vi "VI Tree.vi"   [LabVIEW 2016, in "APT 300XAC Series.lvlib"]
doc: "This instrument driver supports the Associated Power Technologies 300XAC Series Automated AC Power Source\".\n<B>Model Number</B> : 310XAC, 320XAC, 340XAC, 360XAC.\n\nThe VI Tree displays all the user-callable VIs of the instrument driver in an organized table.\n\nAC Range Program mode:\nValue = 0-8; 0=F, 1=A, 2=P, 3=Q, 4=CF, 5=AP, 6=VA, 7=PF, 8=CYCLE\n\nAC Range Manual mode\nValue = 0-7; 0=F, 1=A, 2=P, 3=Q, 4=CF, 5=AP, 6=VA, 7=PF\n\nDC Range Program mode\nValue = 1,2,8; 1=A, 2=P, 8=CYCLE\n\nDC Range Manual mode\nValue = 1,2,8; 1=A, 2=P\n\n\nCreated By:\nAssociated Power Technologies, Inc."
uses:
  APT 300XAC Series.lvlib
  Data/Read Test Data (AC Parallel L1N Program Mode).vi
  Data/Read Test Data (AC Parallel L1N Manual Mode).vi
  Data/Read Step Data (Parallel L1N Manual Mode).vi
  Data/Read Test Data (DC Parallel L1N Program Mode).vi
  Data/Read Test Data (DC Parallel L1N Manual Mode).vi
  Data/Read Step Data (DC Parallel L1N Program Mode).vi
  Data/Read Step Data (DC Parallel L1N Manual Mode).vi
  Data/Read (Voltage).vi
  Data/Read Step Data (AC Total Program Mode).vi
  Data/Read Test Data (AC Program Mode).vi
  Data/Read Step Data (AC Parallel L1N Program Mode).vi
  Data/Read Step Data (AC Polyphase Total Program Mode).vi
  Data/Read Test Data (AC Phase A Program Mode).vi
  Data/Read Test Data (AC Phase A Manual Mode).vi
  Data/Read Step Data (AC Phase A Program Mode).vi
panel:
  # "Associated Power Technologies, Inc. \n1142 S. Diamond Bar Blvd # 106 \nDiamond Bar , CA 91765 \n\nToll Free:  1-877-322-7693\nPhone:      1-909-860-1646\nFax:          1-909-860-2727\nEmail:        info@aspowertechnologies.com"
  # "Please see diagram for APT300XAC Driver VI Tree"
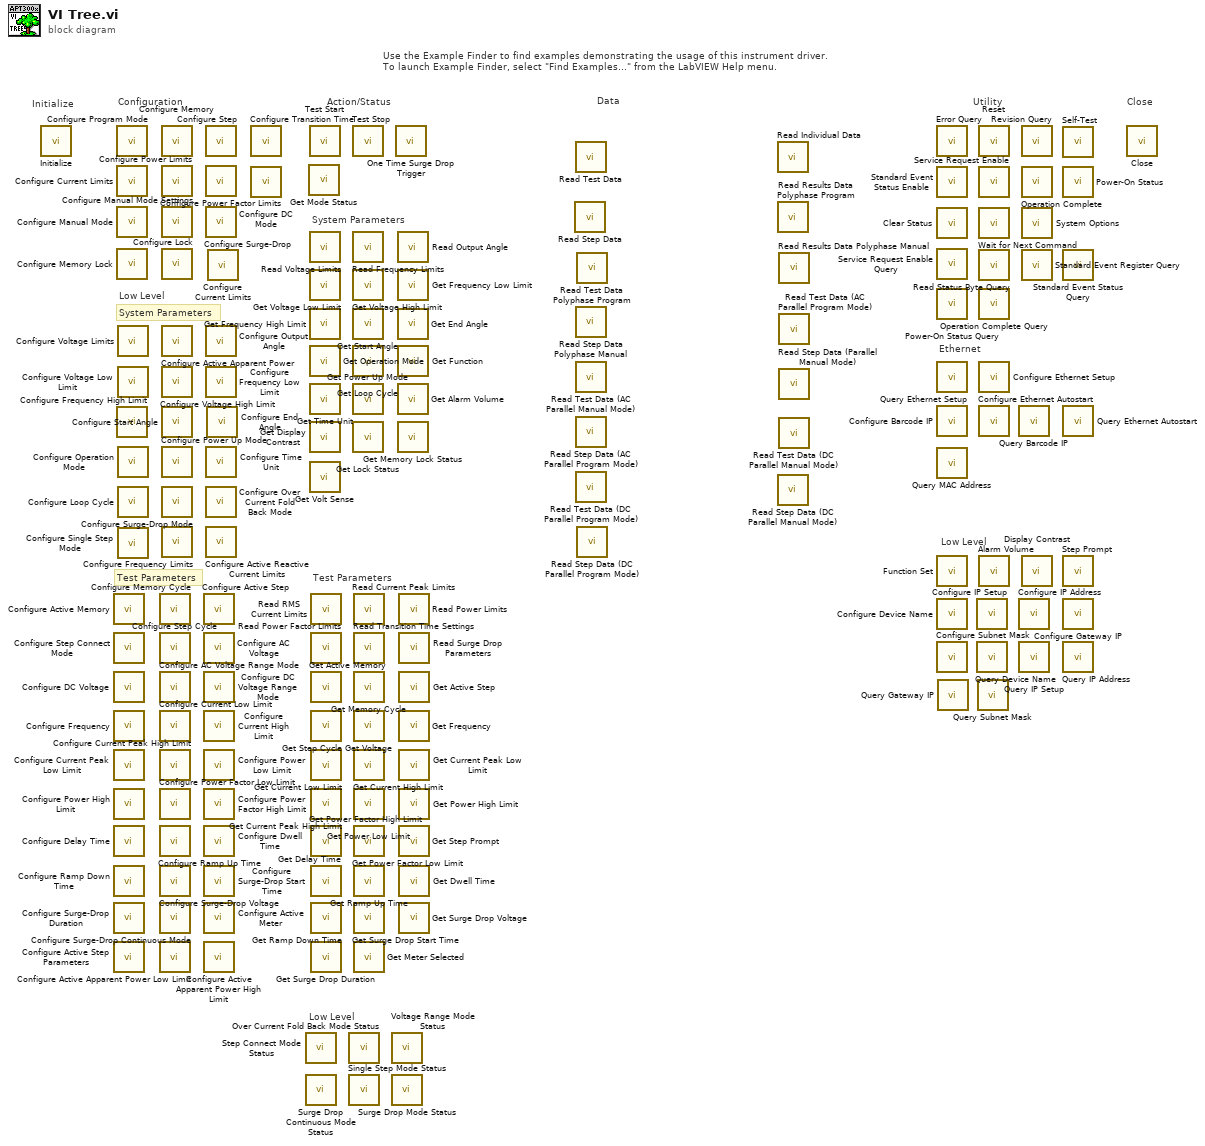
[diagram p0: block diagram]
diagram:
  # "Test Parameters"
  # "System Parameters"
  # "Low Level"
  # "Ethernet"
  # "Low Level"
  # "Use the Example Finder to find examples demonstrating the usage of this instrument driver.\nTo launch Example Finder, select \"Find Examples...\" from the LabVIEW Help menu."
  # "Test Parameters"
  # "System Parameters"
  # "Low Level"
  # "Configuration"
  # "Utility"
  # "Data"
  # "Action/Status"
  # "Close"
  # "Initialize"
  n1 = call "Initialize.vi"() -> ()  [unwired: 14 in, 2 out]
  n2 = call "Configure Active Memory.vi"() -> ()  [unwired: 14 in, 2 out]
  n3 = call "Configure Step Connect Mode.vi"() -> ()  [unwired: 14 in, 2 out]
  n4 = call "Configure DC Voltage.vi"() -> ()  [unwired: 14 in, 2 out]
  n5 = call "Configure Frequency.vi"() -> ()  [unwired: 14 in, 2 out]
  n6 = call "Configure Current Peak Low Limit.vi"() -> ()  [unwired: 14 in, 2 out]
  n7 = call "Configure Power High Limit.vi"() -> ()  [unwired: 14 in, 2 out]
  n8 = call "Configure Delay Time.vi"() -> ()  [unwired: 14 in, 2 out]
  n9 = call "Configure Ramp Down Time.vi"() -> ()  [unwired: 14 in, 2 out]
  n10 = call "Configure Surge-Drop Duration.vi"() -> ()  [unwired: 14 in, 2 out]
  n11 = call "Configure Active Step Parameters.vi"() -> ()  [unwired: 14 in, 2 out]
  n12 = call "Configure Program Mode.vi"() -> ()  [unwired: 14 in, 2 out]
  n13 = call "Configure Current Limits.vi"() -> ()  [unwired: 14 in, 2 out]
  n14 = call "Configure Manual Mode.vi"() -> ()  [unwired: 14 in, 2 out]
  n15 = call "Configure Memory Lock.vi"() -> ()  [unwired: 14 in, 2 out]
  n16 = call "Configure Frequency High Limit.vi"() -> ()  [unwired: 14 in, 2 out]
  n17 = call "Configure Voltage Limits.vi"() -> ()  [unwired: 14 in, 2 out]
  n18 = call "Configure Voltage Low Limit.vi"() -> ()  [unwired: 14 in, 2 out]
  n19 = call "Configure Operation Mode.vi"() -> ()  [unwired: 14 in, 2 out]
  n20 = call "Configure Loop Cycle.vi"() -> ()  [unwired: 14 in, 2 out]
  n21 = call "Configure Single Step Mode.vi"() -> ()  [unwired: 14 in, 2 out]
  n22 = call "Configure Memory Cycle.vi"() -> ()  [unwired: 14 in, 2 out]
  n23 = call "Configure Step Cycle.vi"() -> ()  [unwired: 14 in, 2 out]
  n24 = call "Configure AC Voltage Range Mode.vi"() -> ()  [unwired: 14 in, 2 out]
  n25 = call "Configure Current Low Limit.vi"() -> ()  [unwired: 14 in, 2 out]
  n26 = call "Configure Current Peak High Limit.vi"() -> ()  [unwired: 14 in, 2 out]
  n27 = call "Configure Power Factor Low Limit.vi"() -> ()  [unwired: 14 in, 2 out]
  n28 = call "Configure Ramp Up Time.vi"() -> ()  [unwired: 14 in, 2 out]
  n29 = call "Configure Surge-Drop Voltage.vi"() -> ()  [unwired: 14 in, 2 out]
  n30 = call "Configure Surge-Drop Continuous Mode.vi"() -> ()  [unwired: 14 in, 2 out]
  n31 = call "Configure Active Apparent Power Low Limit.vi"() -> ()  [unwired: 14 in, 2 out]
  n32 = call "Configure Memory.vi"() -> ()  [unwired: 14 in, 2 out]
  n33 = call "Configure Power Limits.vi"() -> ()  [unwired: 14 in, 2 out]
  n34 = call "Configure Manual Mode Settings.vi"() -> ()  [unwired: 14 in, 2 out]
  n35 = call "Configure Lock.vi"() -> ()  [unwired: 14 in, 2 out]
  n36 = call "Configure Active Apparent Power.vi"() -> ()  [unwired: 14 in, 2 out]
  n37 = call "Configure Voltage High Limit.vi"() -> ()  [unwired: 14 in, 2 out]
  n38 = call "Configure Start Angle.vi"() -> ()  [unwired: 14 in, 2 out]
  n39 = call "Configure Power Up Mode.vi"() -> ()  [unwired: 14 in, 2 out]
  n40 = call "Configure Surge-Drop Mode.vi"() -> ()  [unwired: 14 in, 2 out]
  n41 = call "Configure Frequency Limits.vi"() -> ()  [unwired: 14 in, 2 out]
  n42 = call "Configure Active Step.vi"() -> ()  [unwired: 14 in, 2 out]
  n43 = call "Configure AC Voltage.vi"() -> ()  [unwired: 14 in, 2 out]
  n44 = call "Configure DC Voltage Range Mode.vi"() -> ()  [unwired: 14 in, 2 out]
  n45 = call "Configure Current High Limit.vi"() -> ()  [unwired: 14 in, 2 out]
  n46 = call "Configure Power Low Limit.vi"() -> ()  [unwired: 14 in, 2 out]
  n47 = call "Configure Power Factor High Limit.vi"() -> ()  [unwired: 14 in, 2 out]
  n48 = call "Configure Dwell Time.vi"() -> ()  [unwired: 14 in, 2 out]
  n49 = call "Configure Surge-Drop Start Time.vi"() -> ()  [unwired: 14 in, 2 out]
  n50 = call "Configure Active Meter.vi"() -> ()  [unwired: 14 in, 2 out]
  n51 = call "Configure Active Apparent Power High Limit.vi"() -> ()  [unwired: 14 in, 2 out]
  n52 = call "Configure Step.vi"() -> ()  [unwired: 14 in, 2 out]
  n53 = call "Configure Power Factor Limits.vi"() -> ()  [unwired: 14 in, 2 out]
  n54 = call "Configure Surge-Drop.vi"() -> ()  [unwired: 14 in, 2 out]
  n55 = call "Configure Output Angle.vi"() -> ()  [unwired: 14 in, 2 out]
  n56 = call "Configure Frequency Low Limit.vi"() -> ()  [unwired: 14 in, 2 out]
  n57 = call "Configure Time Unit.vi"() -> ()  [unwired: 14 in, 2 out]
  n58 = call "Configure Over Current Fold Back Mode.vi"() -> ()  [unwired: 14 in, 2 out]
  n59 = call "Configure Active Reactive Current Limits.vi"() -> ()  [unwired: 14 in, 2 out]
  n60 = call "Configure End Angle.vi"() -> ()  [unwired: 14 in, 2 out]
  n61 = call "Configure Current Limits.vi"() -> ()  [unwired: 14 in, 2 out]
  n62 = call "Configure Transition Time.vi"() -> ()  [unwired: 14 in, 2 out]
  n63 = call "Configure DC Mode.vi"() -> ()  [unwired: 14 in, 2 out]
  n64 = call "Step Connect Mode Status.vi"() -> ()  [unwired: 13 in, 3 out]
  n65 = call "Surge Drop Continuous Mode Status.vi"() -> ()  [unwired: 13 in, 3 out]
  n66 = call "Get Mode Status.vi"() -> ()  [unwired: 8 in, 8 out]
  n67 = call "Test Start.vi"() -> ()  [unwired: 14 in, 2 out]
  n68 = call "Read Voltage Limits.vi"() -> ()  [unwired: 12 in, 4 out]
  n69 = call "Get Voltage Low Limit.vi"() -> ()  [unwired: 13 in, 3 out]
  n70 = call "Get Frequency High Limit.vi"() -> ()  [unwired: 13 in, 3 out]
  n71 = call "Get Operation Mode.vi"() -> ()  [unwired: 13 in, 3 out]
  n72 = call "Get Time Unit.vi"() -> ()  [unwired: 13 in, 3 out]
  n73 = call "Get Display Contrast.vi"() -> ()  [unwired: 13 in, 3 out]
  n74 = call "Get Volt Sense.vi"() -> ()  [unwired: 9 in, 3 out]
  n75 = call "Read RMS Current Limits.vi"() -> ()  [unwired: 12 in, 4 out]
  n76 = call "Read Power Factor Limits.vi"() -> ()  [unwired: 12 in, 4 out]
  n77 = call "Get Active Memory.vi"() -> ()  [unwired: 13 in, 3 out]
  n78 = call "Get Step Cycle.vi"() -> ()  [unwired: 13 in, 3 out]
  n79 = call "Get Current Low Limit.vi"() -> ()  [unwired: 13 in, 3 out]
  n80 = call "Get Current Peak High Limit.vi"() -> ()  [unwired: 13 in, 3 out]
  n81 = call "Get Power Factor High Limit.vi"() -> ()  [unwired: 13 in, 3 out]
  n82 = call "Get Delay Time.vi"() -> ()  [unwired: 13 in, 3 out]
  n83 = call "Get Ramp Down Time.vi"() -> ()  [unwired: 13 in, 3 out]
  n84 = call "Get Surge Drop Duration.vi"() -> ()  [unwired: 13 in, 3 out]
  n85 = call "Over Current Fold Back Mode Status.vi"() -> ()  [unwired: 13 in, 3 out]
  n86 = call "Single Step Mode Status.vi"() -> ()  [unwired: 13 in, 3 out]
  n87 = call "Test Stop.vi"() -> ()  [unwired: 14 in, 2 out]
  n88 = call "Read Frequency Limits.vi"() -> ()  [unwired: 12 in, 4 out]
  n89 = call "Get Voltage High Limit.vi"() -> ()  [unwired: 13 in, 3 out]
  n90 = call "Get Start Angle.vi"() -> ()  [unwired: 13 in, 3 out]
  n91 = call "Get Loop Cycle.vi"() -> ()  [unwired: 13 in, 3 out]
  n92 = call "Get Power Up Mode.vi"() -> ()  [unwired: 13 in, 3 out]
  n93 = call "Get Lock Status.vi"() -> ()  [unwired: 13 in, 3 out]
  n94 = call "Read Current Peak Limits.vi"() -> ()  [unwired: 12 in, 4 out]
  n95 = call "Read Transition Time Settings.vi"() -> ()  [unwired: 10 in, 6 out]
  n96 = call "Get Memory Cycle.vi"() -> ()  [unwired: 13 in, 3 out]
  n97 = call "Get Voltage.vi"() -> ()  [unwired: 13 in, 3 out]
  n98 = call "Get Current High Limit.vi"() -> ()  [unwired: 13 in, 3 out]
  n99 = call "Get Power Low Limit.vi"() -> ()  [unwired: 13 in, 3 out]
  n100 = call "Get Power Factor Low Limit.vi"() -> ()  [unwired: 13 in, 3 out]
  n101 = call "Get Ramp Up Time.vi"() -> ()  [unwired: 13 in, 3 out]
  n102 = call "Get Surge Drop Start Time.vi"() -> ()  [unwired: 13 in, 3 out]
  n103 = call "Get Meter Selected.vi"() -> ()  [unwired: 13 in, 3 out]
  n104 = call "Voltage Range Mode Status.vi"() -> ()  [unwired: 13 in, 3 out]
  n105 = call "Surge Drop Mode Status.vi"() -> ()  [unwired: 13 in, 3 out]
  n106 = call "One Time Surge Drop Trigger.vi"() -> ()  [unwired: 14 in, 2 out]
  n107 = call "Read Output Angle.vi"() -> ()  [unwired: 12 in, 4 out]
  n108 = call "Get Frequency Low Limit.vi"() -> ()  [unwired: 13 in, 3 out]
  n109 = call "Get End Angle.vi"() -> ()  [unwired: 13 in, 3 out]
  n110 = call "Get Function.vi"() -> ()  [unwired: 13 in, 3 out]
  n111 = call "Get Alarm Volume.vi"() -> ()  [unwired: 13 in, 3 out]
  n112 = call "Get Memory Lock Status.vi"() -> ()  [unwired: 13 in, 3 out]
  n113 = call "Read Power Limits.vi"() -> ()  [unwired: 12 in, 4 out]
  n114 = call "Read Surge Drop Parameters.vi"() -> ()  [unwired: 11 in, 5 out]
  n115 = call "Get Active Step.vi"() -> ()  [unwired: 13 in, 3 out]
  n116 = call "Get Frequency.vi"() -> ()  [unwired: 13 in, 3 out]
  n117 = call "Get Current Peak Low Limit.vi"() -> ()  [unwired: 13 in, 3 out]
  n118 = call "Get Power High Limit.vi"() -> ()  [unwired: 13 in, 3 out]
  n119 = call "Get Step Prompt.vi"() -> ()  [unwired: 13 in, 3 out]
  n120 = call "Get Dwell Time.vi"() -> ()  [unwired: 13 in, 3 out]
  n121 = call "Get Surge Drop Voltage.vi"() -> ()  [unwired: 13 in, 3 out]
  n122 = call-poly "Read Step Data.vi"() -> ()  [unwired: 13 in, 3 out]
  n123 = call-poly "Read Test Data.vi"() -> ()  [unwired: 13 in, 3 out]
  n124 = call-poly "Read Step Data Polyphase Manual.vi"() -> ()  [unwired: 13 in, 3 out]
  n125 = call-poly "Read Test Data (AC Parallel Manual Mode).vi"() -> ()  [unwired: 13 in, 3 out]
  n126 = call-poly "Read Step Data (AC Parallel Program Mode).vi"() -> ()  [unwired: 13 in, 3 out]
  n127 = call-poly "Read Test Data (DC Parallel Program Mode).vi"() -> ()  [unwired: 13 in, 3 out]
  n128 = call-poly "Read Test Data Polyphase Program.vi"() -> ()  [unwired: 13 in, 3 out]
  n129 = call-poly "Read Step Data (DC Parallel Program Mode).vi"() -> ()  [unwired: 13 in, 3 out]
  n130 = call-poly "Read Individual Data.vi"() -> ()  [unwired: 13 in, 3 out]
  n131 = call-poly "Read Results Data Polyphase Program.vi"() -> ()  [unwired: 13 in, 3 out]
  n132 = call-poly "Read Step Data (DC Parallel Manual Mode).vi"() -> ()  [unwired: 13 in, 3 out]
  n133 = call-poly "Read Results Data Polyphase Manual.vi"() -> ()  [unwired: 13 in, 3 out]
  n134 = call-poly "Read Test Data (AC Parallel Program Mode).vi"() -> ()  [unwired: 13 in, 3 out]
  n135 = call-poly "Read Step Data (Parallel Manual Mode).vi"() -> ()  [unwired: 13 in, 3 out]
  n136 = call-poly "Read Test Data (DC Parallel Manual Mode).vi"() -> ()  [unwired: 13 in, 3 out]
  n137 = call "Error Query.vi"() -> ()  [unwired: 12 in, 4 out]
  n138 = call "Standard Event Status Enable.vi"() -> ()  [unwired: 14 in, 2 out]
  n139 = call "Clear Status.vi"() -> ()  [unwired: 14 in, 2 out]
  n140 = call "Service Request Enable Query.vi"() -> ()  [unwired: 13 in, 3 out]
  n141 = call "Power-On Status Query.vi"() -> ()  [unwired: 13 in, 3 out]
  n142 = call "Query Ethernet Setup.vi"() -> ()  [unwired: 5 in, 7 out]
  n143 = call "Configure Barcode IP.vi"() -> ()  [unwired: 14 in, 2 out]
  n144 = call "Query MAC Address.vi"() -> ()  [unwired: 13 in, 3 out]
  n145 = call "Function Set.vi"() -> ()  [unwired: 14 in, 2 out]
  n146 = call "Configure Device Name.vi"() -> ()  [unwired: 14 in, 2 out]
  n147 = call "Configure Subnet Mask.vi"() -> ()  [unwired: 14 in, 2 out]
  n148 = call "Query Gateway IP.vi"() -> ()  [unwired: 13 in, 3 out]
  n149 = call "Configure IP Setup.vi"() -> ()  [unwired: 14 in, 2 out]
  n150 = call "Query Device Name.vi"() -> ()  [unwired: 13 in, 3 out]
  n151 = call "Query Subnet Mask.vi"() -> ()  [unwired: 13 in, 3 out]
  n152 = call "Reset.vi"() -> ()  [unwired: 14 in, 2 out]
  n153 = call "Service Request Enable.vi"() -> ()  [unwired: 14 in, 2 out]
  n154 = call "Wait for Next Command.vi"() -> ()  [unwired: 14 in, 2 out]
  n155 = call "Read Status Byte Query.vi"() -> ()  [unwired: 13 in, 3 out]
  n156 = call "Operation Complete Query.vi"() -> ()  [unwired: 13 in, 3 out]
  n157 = call "Configure Ethernet Setup.vi"() -> ()  [unwired: 10 in, 2 out]
  n158 = call "Configure Ethernet Autostart.vi"() -> ()  [unwired: 14 in, 2 out]
  n159 = call "Alarm Volume.vi"() -> ()  [unwired: 14 in, 2 out]
  n160 = call "Query Barcode IP.vi"() -> ()  [unwired: 13 in, 3 out]
  n161 = call "Configure IP Address.vi"() -> ()  [unwired: 14 in, 2 out]
  n162 = call "Query IP Setup.vi"() -> ()  [unwired: 13 in, 3 out]
  n163 = call "Revision Query.vi"() -> ()  [unwired: 11 in, 5 out]
  n164 = call "Operation Complete.vi"() -> ()  [unwired: 14 in, 2 out]
  n165 = call "System Options.vi"() -> ()  [unwired: 10 in, 2 out]
  n166 = call "Standard Event Register Query.vi"() -> ()  [unwired: 13 in, 3 out]
  n167 = call "Display Contrast.vi"() -> ()  [unwired: 14 in, 2 out]
  n168 = call "Self-Test.vi"() -> ()  [unwired: 12 in, 4 out]
  n169 = call "Power-On Status.vi"() -> ()  [unwired: 14 in, 2 out]
  n170 = call "Standard Event Status Query.vi"() -> ()  [unwired: 13 in, 3 out]
  n171 = call "Query Ethernet Autostart.vi"() -> ()  [unwired: 13 in, 3 out]
  n172 = call "Step Prompt.vi"() -> ()  [unwired: 14 in, 2 out]
  n173 = call "Configure Gateway IP.vi"() -> ()  [unwired: 14 in, 2 out]
  n174 = call "Query IP Address.vi"() -> ()  [unwired: 13 in, 3 out]
  n175 = call "Close.vi"() -> ()  [unwired: 15 in, 1 out]
